vi "alias tree dialog.vi"(6 "Tree Config":T2, 7 "SDF Path":path=path "C:/Users/Public/Documents/National Instruments/NI VeriStand 2017/Examples/Stimulus Profile/Engine Demo/Engine Demo.nivssdf", 8 "error in (no error)":errorcluster, 9 "Use AND Logic (F)":bool, 10 "Filter Config":T1(array[cluster]), 11 "Current Selection":string[](array[string])=["Aliases/ActualRPM", "Aliases/DesiredRPM", "Aliases/Engine Calculations/RPM Acceleration", "Aliases/Engine Calculations/RPM Velocity", "Aliases/Engine Calculations/Engine Revolutions", "Aliases/Engine Calculations/RPM Offset", "Aliases/Engine Calculations/RPM Valley", "Aliases/Engine Calculations/RPM Peak", "Aliases/Engine Calculations/RPM Set Point Difference", "Aliases/Engine Safety Limits/Engine Temperature Alert", "Aliases/Engine Safety Limits/Engine Temperature Warning", "Aliases/EnginePower", "Aliases/EngineTemp", "Aliases/Idle Speed"]) -> (0 "error out":errorcluster, 3 "Selected Paths":string[](array[string])=["Aliases/ActualRPM", "Aliases/DesiredRPM", "Aliases/Engine Calculations/RPM Acceleration", "Aliases/Engine Calculations/RPM Velocity", "Aliases/Engine Calculations/Engine Revolutions", "Aliases/Engine Calculations/RPM Offset", "Aliases/Engine Calculations/RPM Valley", "Aliases/Engine Calculations/RPM Peak", "Aliases/Engine Calculations/RPM Set Point Difference", "Aliases/Engine Safety Limits/Engine Temperature Alert", "Aliases/Engine Safety Limits/Engine Temperature Warning", "Aliases/EnginePower", "Aliases/EngineTemp", "Aliases/Idle Speed"])   [LabVIEW 2017, in "vs-tree-utility.lvlib"]
uses:
  alias-tree/methods/set filter (channel).vi
  alias-tree/methods/set filter (waveform).vi
  alias-tree/methods/set filter (section).vi
  alias-tree/methods/set current selection (multiple).vi
  alias-tree/alias-tree.lvclass
  vs-tree-utility.lvlib
  NationalInstruments.VeriStand.SystemStorageUI
panel:
  in  "TreeAliasBrowserWF":refnum<k24>(container)
  in  "Stop":bool
  # "Text here"
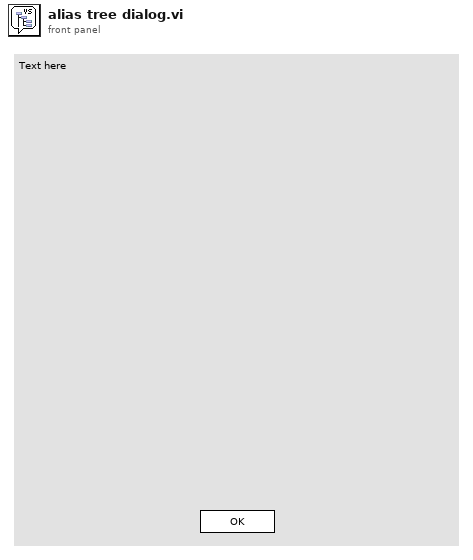
[diagram p1: front panel]
types:
  T1 = cluster{"Type":enum16{"Channel", "Waveform", "Section"}, "Parameters":variant, "Show Only Visible?":bool}[]
  T2 = cluster{"Allow Multi Select":bool, "Use Checkboxes":bool, "Text Prompt":string}
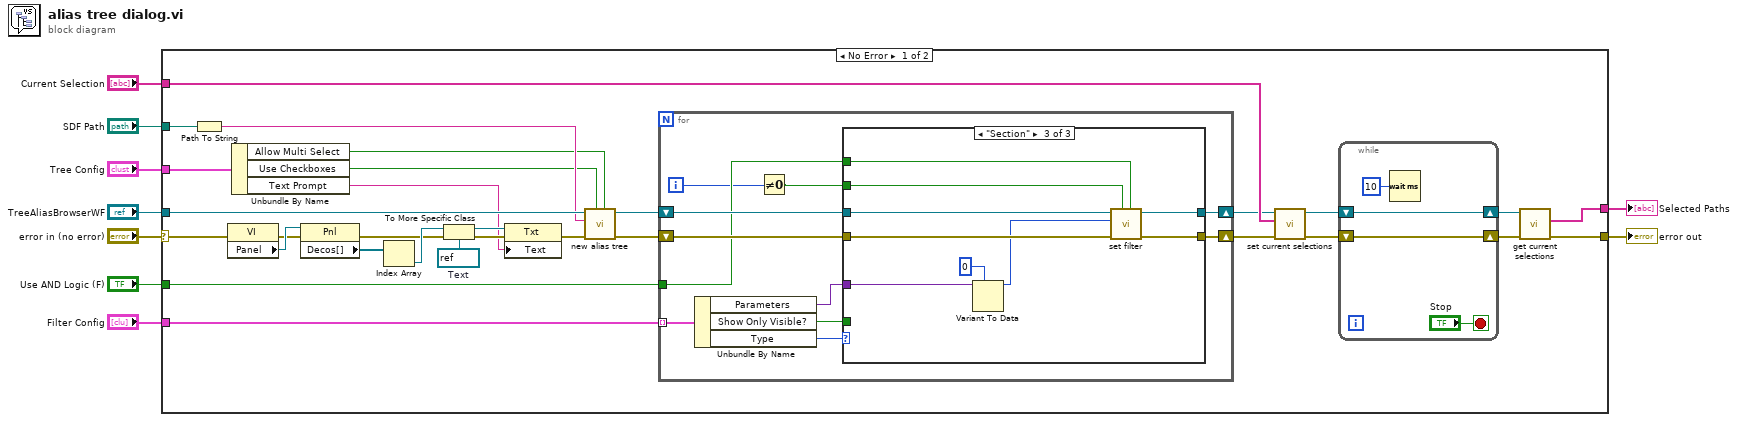
[diagram p0: block diagram]
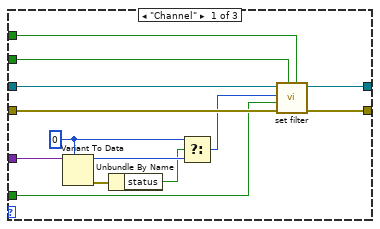
[diagram p2: hidden frame]
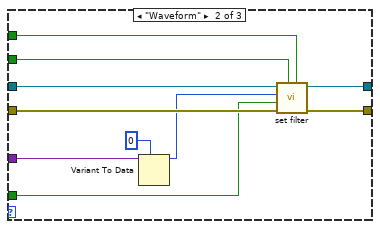
[diagram p3: hidden frame]
diagram:
  n1 = case shown="No Error" "error in (no error)" {
    selector: "error in (no error)" -> [w16 w87]
    tunnel: "TreeAliasBrowserWF" -> [w39 _]
    tunnel: "SDF Path" -> [w38 _]
    tunnel: "Current Selection" -> [w33 _]
    tunnel: [w22 _] -> w6
    tunnel: "Tree Config" -> [w20 _]
    tunnel: [w15 w87] -> w3
    tunnel: "Filter Config" -> [w11 _]
    tunnel: "Use AND Logic (F)" -> [w10 _]
    frame No Error {
      w25 = refnum<vi> refnum  # Text
      n2 = Path To String(path=w38) -> (string=w37:string)
      n3 = property class="VI"(error in=w16) -> (error out=w27:errorcluster, "Panel"=w30:refnum<vi>)  [unwired: 1 in, 1 out]
      n4 = Unbundle By Name(w20) -> ("Allow Multi Select"=w19:bool, "Use Checkboxes"=w18:bool, "Text Prompt"=w17:string)
      n5 = property class="Pnl"(reference=w30, error in=w27) -> (error out=w26:errorcluster, "Decos[]"=w29:refnum<vi>[])  [unwired: 1 out]
      n6 = Index Array(array=w29) -> (element=w28:refnum<vi>)  [unwired: 1 in]
      n7 = To More Specific Class(target class=w25, reference=w28, error in=w26) -> (specific class reference=w24:refnum<vi>, error out=w23:errorcluster)
      n8 = property class="Txt"(reference=w24, error in=w23, "Text"=w17) -> (error out=w21:errorcluster)  [unwired: 1 out]
      n9 = call "new alias tree.vi"("allow multi-select"=w19, "show checkbox"=w18, "error in (no error)"=w21, "sdf path"=w37, "tree ref"=w39) -> ("error out"=w36:errorcluster, "alias-tree"=w13:refnum<class "alias-tree.lvclass">)  [unwired: 5 in]
      n10 = for {
        shift-right: [w49] -> w14
        shift-left: w36 -> [w50]
        shift-right: [w47] -> w12
        shift-left: w13 -> [w48]
        tunnel: w11 -> [w46] mode=indexing
        tunnel: w10 -> [w44]
        i -> [w41]
        n11 = Unbundle By Name(w46) -> ("Parameters"=w43:variant, "Show Only Visible?"=w45:bool, "Type"=w42:enum16{"Channel", "Waveform", "Section"})
        n12 = Not Equal To 0?(x=w41) -> (x != 0?=w40:bool)
        n13 = case shown="\"Section\"" w42 {
          tunnel: w50 -> [w63 w73 w82]
          tunnel: [w62 w72 w81] -> w49
          tunnel: w48 -> [w61 w71 w80]
          tunnel: [w60 w70 w79] -> w47
          tunnel: w44 -> [w59 w69 w78]
          tunnel: w43 -> [w57 w67 w77]
          tunnel: w45 -> [w58 w68 _]
          tunnel: w40 -> [w51 w64 w74]
          frame "Channel" {
            w55 = u16 0
            n14 = Variant To Data(type=w55, Variant=w57) -> (data=w56:u16, error out=w54:errorcluster)  [unwired: 1 in]
            n15 = Unbundle By Name(w54) -> ("status"=w53:bool)
            n16 = Select(t=w55, s=w53, f=w56) -> (s? t:f=w52:u16)
            n17 = call-poly "set filter.vi"("Use AND Logic? (False)"=w59, "Combine Existing (False)"=w51, "error in (no error)"=w63, "Include Only Visible?"=w58, "Type"=w52, "alias-tree in"=w61) -> ("error out"=w62:errorcluster, "alias-tree out"=w60:refnum<class "alias-tree.lvclass">)  [unwired: 4 in]
          }
          frame "Waveform" {
            n18 = Variant To Data(type=u16 0, Variant=w67) -> (data=w65:u16)  [unwired: 1 in, 1 out]
            n19 = call-poly "set filter.vi"("Use AND Logic? (False)"=w69, "Combine Existing (False)"=w64, "error in (no error)"=w73, "Include Only Visible?"=w68, "Type"=w65, "alias-tree in"=w71) -> ("error out"=w72:errorcluster, "alias-tree out"=w70:refnum<class "alias-tree.lvclass">)  [unwired: 4 in]
          }
          frame "Section" {
            n20 = Variant To Data(type=u16 0, Variant=w77) -> (data=w75:u16)  [unwired: 1 in, 1 out]
            n21 = call-poly "set filter.vi"("Use AND Logic? (False)"=w78, "Combine Existing (False)"=w74, "error in (no error)"=w82, "Type"=w75, "alias-tree in"=w80) -> ("error out"=w81:errorcluster, "alias-tree out"=w79:refnum<class "alias-tree.lvclass">)  [unwired: 5 in]
          }
        }
      }
      n22 = call-poly "set current selections.vi"("error in (no error)"=w14, "paths"=w33, "alias-tree in"=w12) -> ("error out"=w31:errorcluster, "alias-tree out"=w32:refnum<class "alias-tree.lvclass">)  [unwired: 5 in, 2 out]
      n23 = while {
        shift-right: [w83] -> w35
        shift-left: w32 -> [w83]
        shift-right: [w84] -> w34
        shift-left: w31 -> [w84]
        stop <- "Stop" stop-if-true
        n24 = Wait (ms)(milliseconds to wait=u32 10) -> ()  [unwired: 1 out]
      }
      n25 = call-dynamic "get current selections.vi"("error in (no error)"=w34, "Tree in"=w35) -> ("error out"=w15:errorcluster, "Selected Paths"=w22:string[])  [unwired: 7 in, 1 out]
    }
    frame Error {
    }
  }
  "Selected Paths" <- w6
  "error out" <- w3
